vi "Generate txt Report.vi"(0 "Serial Number":string, 1 "Testing result":string, 2 "Failed Tests":string, 3 "Upper Limits":dbl[](array[numeric]), 4 "Lower Limits":dbl[](array[numeric]), 5 "Measurement values":dbl[](array[numeric]), 6 "Test Names":string[](array[string]), 7 "Status":string[](array[string]), 9 "NTC Codes":string) -> (14 "Critical NTC":bool, 15 "Fault NTC":bool, 19 "error out":errorcluster)   [LabVIEW 2025]
uses:
  <vilib>/Utility/file.llb/Read Delimited Spreadsheet (string).vi
  <vilib>/Utility/file.llb/Write Delimited Spreadsheet (string).vi
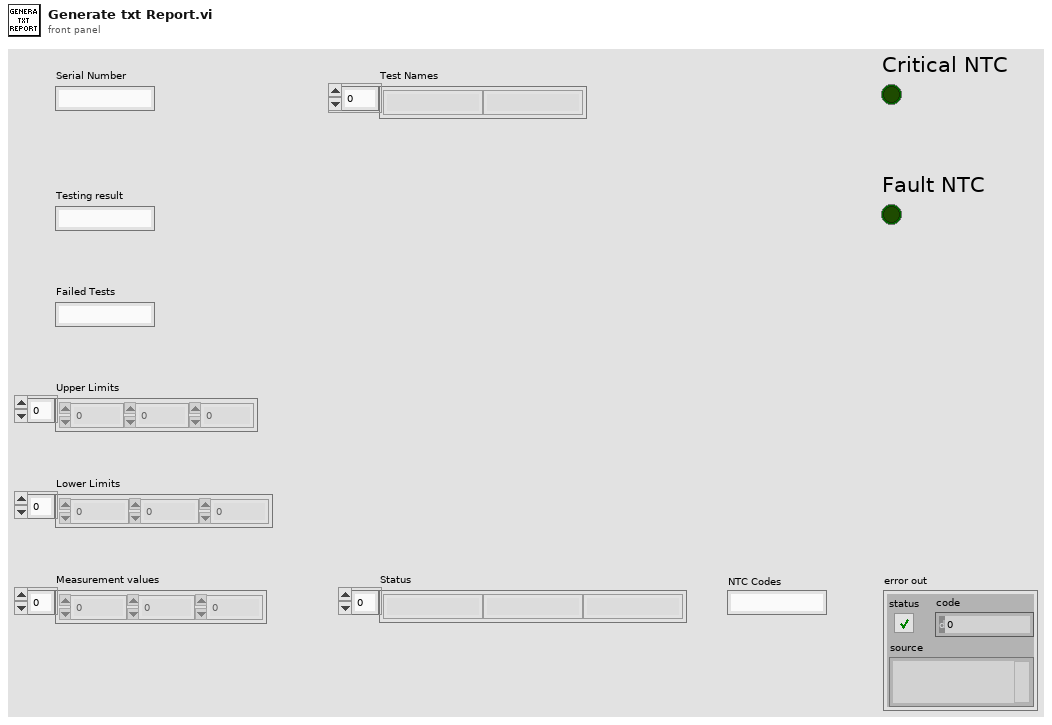
[diagram p1: front panel]
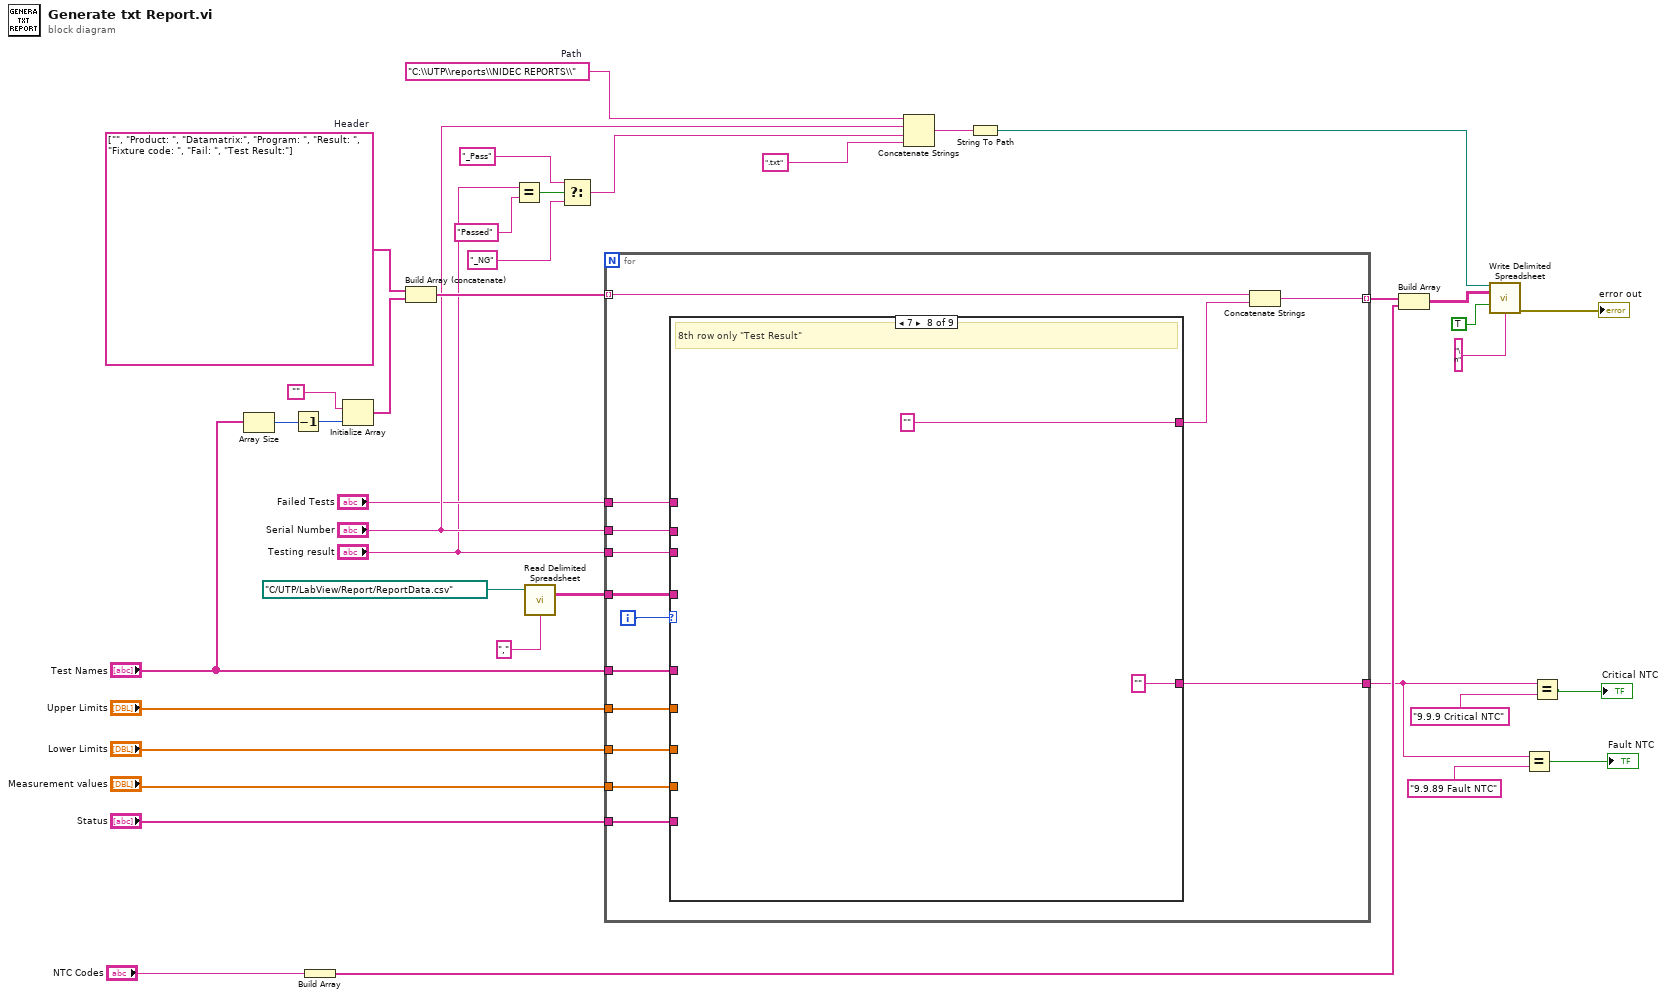
[diagram p0: block diagram]
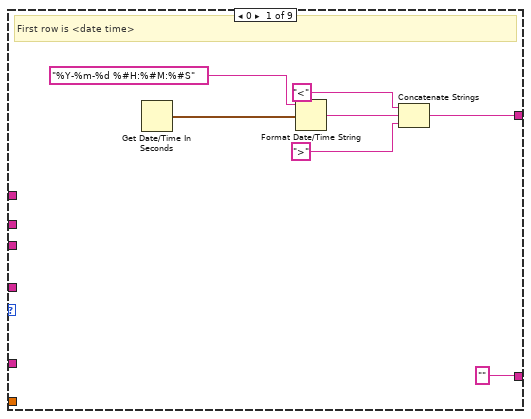
[diagram p2: hidden frame]
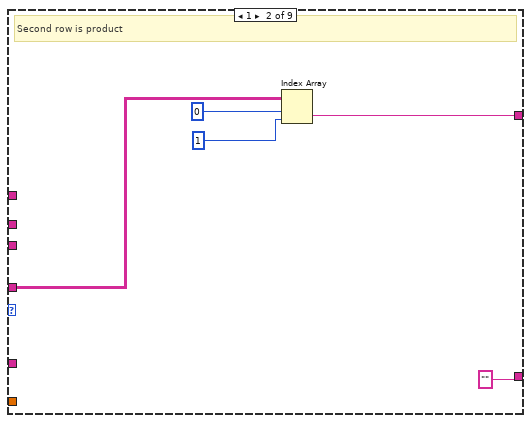
[diagram p3: hidden frame]
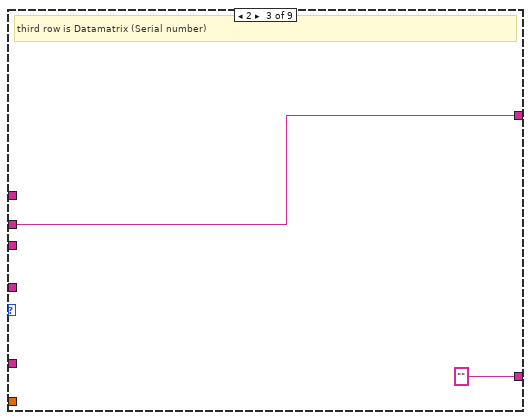
[diagram p4: hidden frame]
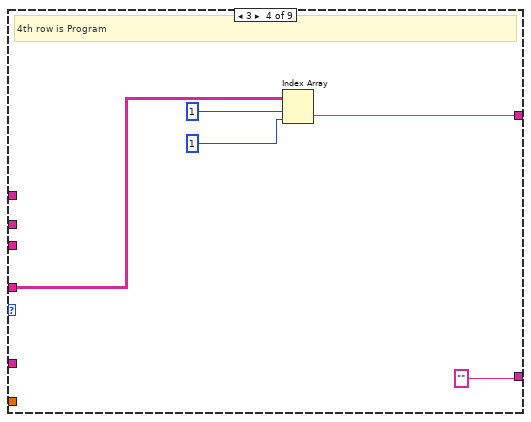
[diagram p5: hidden frame]
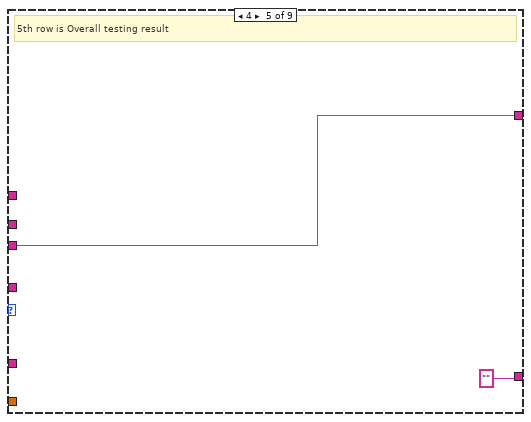
[diagram p6: hidden frame]
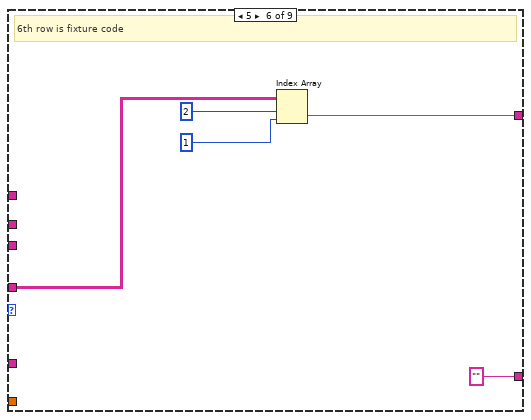
[diagram p7: hidden frame]
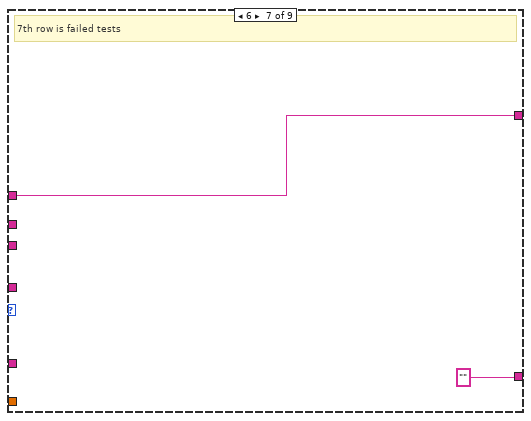
[diagram p8: hidden frame]
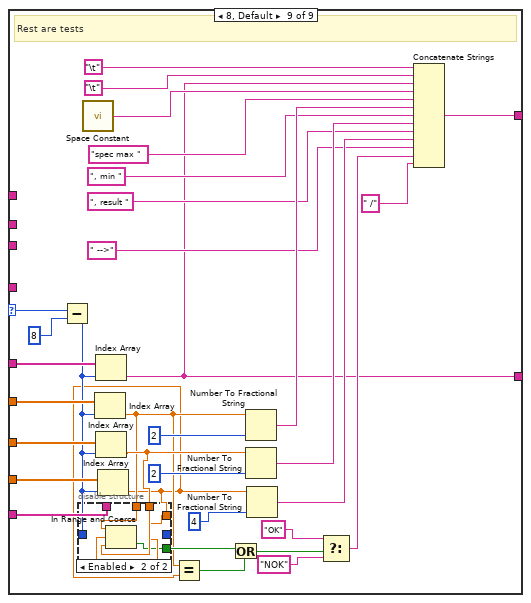
[diagram p9: hidden frame]
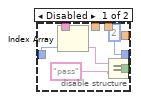
[diagram p10: hidden frame]
diagram:
  w33 = "C:\\UTP\\reports\\NIDEC REPORTS\\"  # Path
  w24 = string[] ["", "Product: ", "Datamatrix:", "Program: ", "Result: ", "Fixture code: ", "Fail: ", "Test Result:"]  # Header
  n1 = Array Size(array="Test Names") -> (size(s)=w27:i32)
  n2 = Decrement(x=w27) -> (x-1=w10:i32)
  n3 = Build Array("NTC Codes") -> (w6:string[])
  n4 = Initialize Array("", w10) -> (w25:string[])
  n5 = Build Array (concatenate)(w24, w25) -> (w21:string[])
  n6 = Equal?(x="Testing result", y="Passed") -> (x = y?=w15:bool)
  n7 = call-poly <vilib>:"Read Delimited Spreadsheet.vi"("file path (dialog if empty)"=path "C:/UTP/LabView/Report/ReportData.csv", "delimiter (\\t)"="," ("delimiter (\\t)")) -> ("all rows"=w20:string[][])  [unwired: 8 in, 5 out]
  n8 = Select(t="_Pass" ("y"), s=w15, f="_NG") -> (s? t:f=w12:string)
  n9 = for {
    tunnel: "Upper Limits" -> [w47]
    tunnel: "Lower Limits" -> [w46]
    tunnel: "Measurement values" -> [w45]
    tunnel: "Status" -> [w44]
    tunnel: "Test Names" -> [w48]
    tunnel: w21 -> [w42] mode=indexing
    tunnel: [w40] -> w9 mode=indexing
    tunnel: w20 -> [w51]
    tunnel: "Serial Number" -> [w50]
    tunnel: "Testing result" -> [w49]
    tunnel: "Failed Tests" -> [w43]
    tunnel: [w39] -> w1
    i -> [w52]
    n10 = case shown="7" w52 {
      selector: w52 -> [_ _ _ _ _ _ _ _ w110]
      tunnel: [w54 w61 w66 w68 w73 w75 w80 "" ("Failed Tests") w92] -> w41
      tunnel: w51 -> [_ w64 _ w69 _ w76 _ _ _]
      tunnel: w50 -> [_ _ w66 _ _ _ _ _ _]
      tunnel: w49 -> [_ _ _ _ w73 _ _ _ _]
      tunnel: w48 -> [_ _ _ _ _ _ _ _ w115]
      tunnel: w47 -> [_ _ _ _ _ _ _ _ w114]
      tunnel: w46 -> [_ _ _ _ _ _ _ _ w113]
      tunnel: w45 -> [_ _ _ _ _ _ _ _ w112]
      tunnel: w44 -> [_ _ _ _ _ _ _ _ w111]
      tunnel: w43 -> [_ _ _ _ _ _ w80 _ _]
      tunnel: ["" ("Test Names") "" ("Test Names") "" ("Test Names") "" ("Test Names") "" ("Test Names") "" ("Test Names") "" ("Test Names") "" ("Test Names") w83] -> w39
      frame 0 {
        # "First row is <date time>"
        n11 = Get Date/Time In Seconds() -> (seconds since 1Jan1904=w59:timestamp)
        n12 = Format Date/Time String(time format string (%c)="%Y-%m-%d %#H:%#M:%#S", seconds (now)=w59) -> (date/time string=w58:string)  [unwired: 1 in]
        n13 = Concatenate Strings("<" ("string"), w58, ">" ("string")) -> (w54:string)
      }
      frame 1 {
        # "Second row is product"
        n14 = Index Array(array=w64, index (row)=0, index (col)=1) -> (element=w61:string)
      }
      frame 2 {
        # "third row is Datamatrix (Serial number)"
      }
      frame 3 {
        # "4th row is Program"
        n15 = Index Array(array=w69, index (row)=1, index (col)=1) -> (element=w68:string)
      }
      frame 4 {
        # "5th row is Overall testing result"
      }
      frame 5 {
        # "6th row is fixture code"
        n16 = Index Array(array=w76, index (row)=2, index (col)=1) -> (element=w75:string)
      }
      frame 6 {
        # "7th row is failed tests"
      }
      frame 7 {
        # "8th row only \"Test Result\""
      }
      frame 8, Default {
        # "Rest are tests"
        n17 = Subtract(x=w110, y=8) -> (x-y=w108:i32)
        n18 = call <vilib>:"Space Constant.vi"() -> ("String"=w103:string)
        n19 = Index Array(array=w114, index=w108) -> (element=w88:dbl)
        n20 = Index Array(array=w115, index=w108) -> (element=w83:string)
        n21 = Index Array(array=w113, index=w108) -> (element=w90:dbl)
        n22 = Index Array(array=w112, index=w108) -> (element=w87:dbl)
        n23 = disable-structure shown="Enabled" {
          disable-tunnel: [i16 2 ("precision (6)") _] -> _
          disable-tunnel: w111 -> [w120 _]
          disable-tunnel: w108 -> [w119 _]
          disable-tunnel: [w116 w122] -> w89
          disable-tunnel: w88 -> [_ w125]
          disable-tunnel: w90 -> [_ w124]
          disable-tunnel: w87 -> [_ w123]
          frame Disabled {
            n24 = Index Array(array=w120, index=w119) -> (element=w118:string)
            n25 = Equal?(x=w118, y="pass") -> (x = y?=w116:bool)
          }
          frame Enabled {
            n26 = In Range and Coerce(upper limit=w125, x=w123, lower limit=w124) -> (In Range?=w122:bool)  [unwired: 1 out]
          }
        }
        n27 = Equal?(x=w88, y=w87) -> (x = y?=w86:bool)
        n28 = Or(x=w89, y=w86) -> (x .or. y?=w85:bool)
        n29 = Number To Fractional String(number=w88, precision (6)=i16 2) -> (F-format string=w101:string)  [unwired: 2 in]
        n30 = Number To Fractional String(number=w90, precision (6)=i16 2) -> (F-format string=w99:string)  [unwired: 2 in]
        n31 = Number To Fractional String(number=w87, precision (6)=i16 4) -> (F-format string=w97:string)  [unwired: 2 in]
        n32 = Select(t="OK" ("y"), s=w85, f="NOK" ("y")) -> (s? t:f=w93:string)
        n33 = Concatenate Strings("\t", "\t", w83, w103, "spec max " ("string"), w101, ", min " ("string"), w99, ", result " ("string"), w97, " -->" ("string"), w93, " /" ("string")) -> (w92:string)
      }
    }
    n34 = Concatenate Strings(w42, w41) -> (w40:string)
  }
  n35 = Concatenate Strings(w33, "Serial Number", w12, ".txt" ("string")) -> (w32:string)
  n36 = String To Path(string=w32) -> (path=w31:path)
  n37 = Build Array(w9, w6) -> (w8:string[][])
  n38 = call-poly <vilib>:"Write Delimited Spreadsheet.vi"("file path (dialog if empty)"=w31, "2D data"=w8, "append to file? (new file:F)"=TRUE, "delimiter (\\t)"="\n" ("delimiter (\\t)")) -> ("error out"=→"error out":errorcluster)  [unwired: 10 in, 1 out]
  n39 = Equal?(x=w1, y="9.9.89 Fault NTC") -> (x = y?=→"Fault NTC":bool)
  n40 = Equal?(x=w1, y="9.9.9 Critical NTC") -> (x = y?=→"Critical NTC":bool)
